vi "FindSubpanels.PathArray.vi"(6 "Append (F)":bool, 8 "error in":errorcluster, 10 "Subpanel List":path[](array[path]), 11 "SMO.UI.MAUI in":refnum<class "SMO.UI.MAUI.lvclass">) -> (0 "error out":errorcluster, 3 "SMO.UI.MAUI out":refnum<class "SMO.UI.MAUI.lvclass">)   [LabVIEW 2019, in "SMO.UI.MAUI.lvclass"]
uses:
  SMO.UI.MAUI.lvclass
  <vilib>/JKI/JKI SMO/SMO/SMO.lvclass
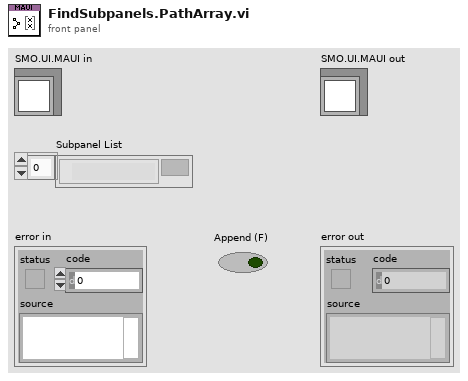
[diagram p1: front panel]
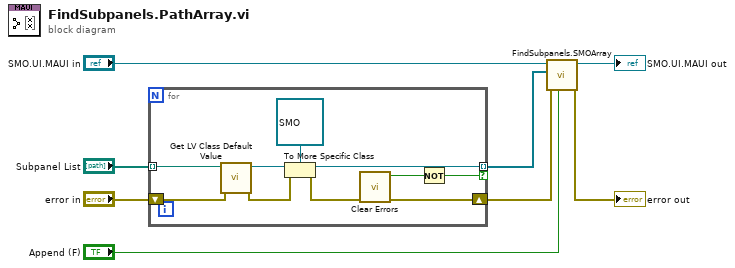
[diagram p0: block diagram]
diagram:
  n1 = for {
    tunnel: "Subpanel List" -> [w18] mode=indexing
    tunnel: [w15] -> w2 mode=indexing if=w13
    shift-right: [w11] -> w1
    shift-left: "error in" -> [w10]
    n2 = call <vilib>:"Get LV Class Default Value.vi"("error in (no error)"=w10, "class path"=w18) -> ("error out"=w16:errorcluster, "object"=w17:refnum<class>)  [unwired: 8 in]
    n3 = To More Specific Class(target class=refnum<class "SMO.lvclass"> refnum ("SMO"), reference=w17, error in=w16) -> (specific class reference=w15:refnum<class "SMO.lvclass">, error out=w14:errorcluster)
    n4 = call <vilib>:"Clear Errors.vi"("error in (no error)"=w14) -> ("error out"=w11:errorcluster, "specific error cleared?"=w12:bool)  [unwired: 5 in]
    n5 = Not(x=w12) -> (.not. x?=w13:bool)
  }
  n6 = call-dynamic "FindSubpanels.SMOArray.vi"("Append (F)"="Append (F)", "error in"=w1, "Subpanels"=w2, "SMO.UI.MAUI in"="SMO.UI.MAUI in") -> ("error out"=→"error out":errorcluster, "SMO.UI.MAUI out"=→"SMO.UI.MAUI out":refnum<class "SMO.UI.MAUI.lvclass">)  [unwired: 6 in]
